vi "smgrIO.vi"(3 "error IO 2":errorcluster, 4 "URL":string, 5 "Array":T1[](array[typedef])) -> (0 "error IO":errorcluster, 1 "body":string, 2 "headers":string)   [LabVIEW 2010]
uses:
  <vilib>/httpClient/MultipartData.ctl
  <vilib>/httpClient/LabVIEWHTTPClient.lvlib
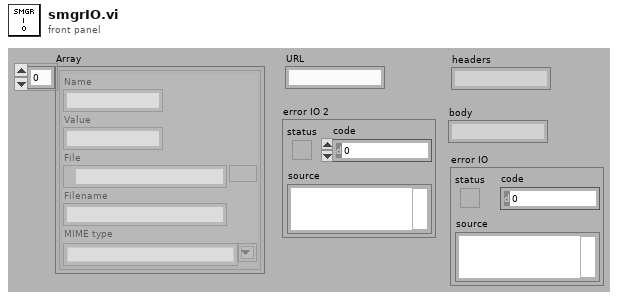
[diagram p1: front panel]
types:
  T1 = typedef "LabVIEWHTTPClient.lvlib/MultipartData.ctl" = cluster{"Name":string, "Value":string, "File":path, "Filename":string, "MIME type":string}
  T2 = typedef "LabVIEWHTTPClient.lvlib/ClientHandle.ctl" = refnum<k1>
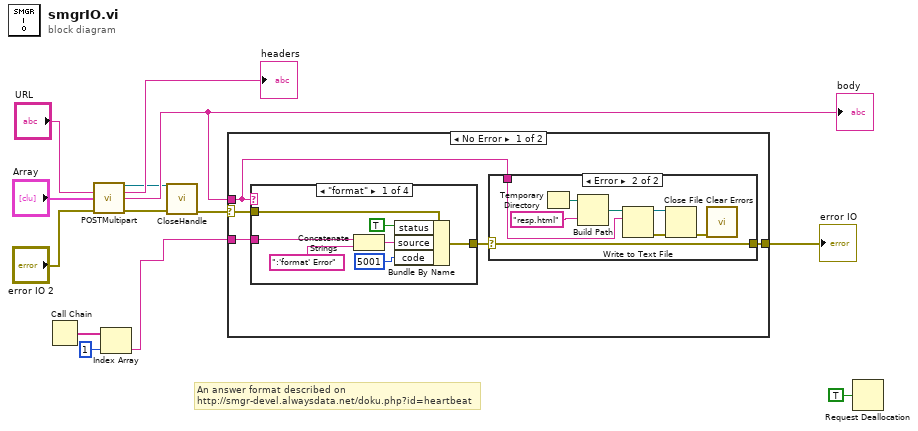
[diagram p0: block diagram]
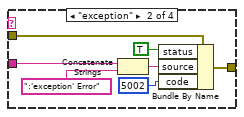
[diagram p3: hidden frame]
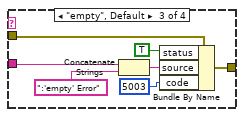
[diagram p4: hidden frame]
diagram:
  # "An answer format described on\nhttp://smgr-devel.alwaysdata.net/doku.php?id=heartbeat"
  n1 = Call Chain() -> (call chain=w4:string[])
  n2 = call <vilib>:"POSTMultipart.vi"("URL"="URL", "data"="Array", "error in (no error)"="error IO 2") -> ("client handle out"=w6:T2, "headers"=→"headers":string, "body"=w12:string, "error out"=w8:errorcluster)  [unwired: 9 in]
  "body" <- w12
  n3 = Index Array(array=w4, index=1) -> (element=w3:string)
  n4 = call <vilib>:"CloseHandle.vi"("client handle"=w6, "error in (no error)"=w8) -> ("error out"=w11:errorcluster)  [unwired: 13 in]
  n5 = case shown="No Error" w11 {
    selector: w11 -> [w18 w50]
    tunnel: [w14 w50] -> w13
    tunnel: w12 -> [w16 _]
    tunnel: w3 -> [w17 _]
    frame No Error {
      n6 = case shown="\"format\"" w16 {
        tunnel: w18 -> [w32 w36 w44 w49]
        tunnel: [w33 w35 w42 w49] -> w15
        tunnel: w17 -> [w34 w37 w43 _]
        frame "format" {
          n7 = Concatenate Strings(w34, ":'format' Error") -> (w29:string)
          n8 = Bundle By Name(cluster=w32, "status"=TRUE, "source"=w29, "code"=5001) -> (w33:errorcluster)
        }
        frame "exception" {
          n9 = Concatenate Strings(w37, ":'exception' Error") -> (w40:string)
          n10 = Bundle By Name(cluster=w36, "status"=TRUE, "source"=w40, "code"=5002) -> (w35:errorcluster)
        }
        frame "empty", Default {
          n11 = Concatenate Strings(w43, ":'empty' Error") -> (w47:string)
          n12 = Bundle By Name(cluster=w44, "status"=TRUE, "source"=w47, "code"=5003) -> (w42:errorcluster)
        }
        frame "ok" {
        }
      }
      n13 = case shown="Error" w15 {
        selector: w15 -> [w19 w21]
        tunnel: w16 -> [_ w22]
        tunnel: [w19 w21] -> w14
        frame No Error {
        }
        frame Error {
          n14 = Temporary Directory() -> (w27:path)
          n15 = Build Path(base path=w27, name or relative path="resp.html") -> (appended path=w25:path)
          n16 = Write to Text File(file (use dialog)=w25, text=w22) -> (refnum out=w23:refnum<file>, error out=w24:errorcluster)  [unwired: 2 in, 1 out]
          n17 = Close File(refnum=w23, error in=w24) -> (error out=w20:errorcluster)  [unwired: 1 out]
          n18 = call <vilib>:"Clear Errors.vi"("error in (no error)"=w20) -> ()  [unwired: 6 in, 1 out]
        }
      }
    }
    frame Error {
    }
  }
  "error IO" <- w13
  n19 = Request Deallocation(TRUE ("flag")) -> ()
